vi "Conf_DO.vi"(8 "error in (no error)":errorcluster, 10 "PIN Number":i8, 11 "DI_DO in":refnum<class "DI_DO.lvclass">) -> (0 "error out":errorcluster, 3 "DI_DO out":refnum<class "DI_DO.lvclass">)   [LabVIEW 2023, in "Driver_DI_DO.lvlib" / "DI_DO.lvclass"]
uses:
  DI_DO.lvclass
  DI_DO.lvclass/DI_DO.ctl
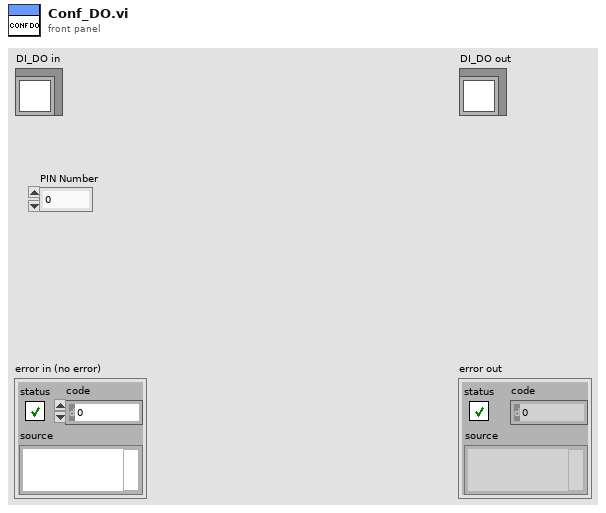
[diagram p1: front panel]
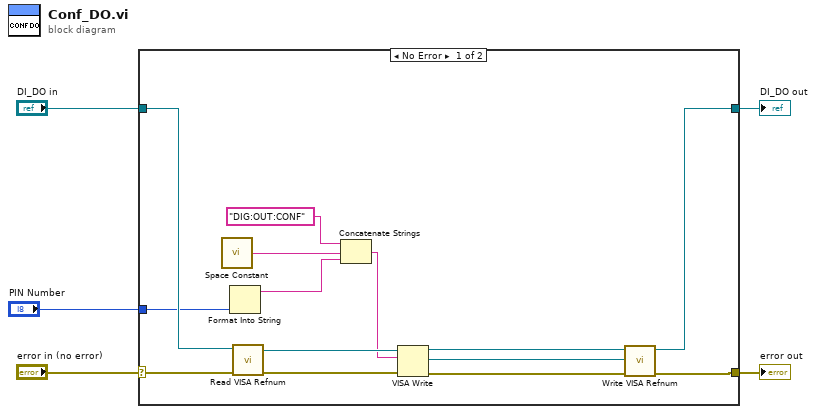
[diagram p0: block diagram]
diagram:
  n1 = case shown="No Error" "error in (no error)" {
    selector: "error in (no error)" -> [w18 w21]
    tunnel: [w9 w21] -> w4
    tunnel: [w7 w20] -> w2
    tunnel: "DI_DO in" -> [w19 w20]
    tunnel: "PIN Number" -> [w17 _]
    frame No Error {
      n2 = call <vilib>:"Space Constant.vi"() -> ("String"=w15:string)
      n3 = Format Into String(w17) -> (resulting string=w14:string)  [unwired: 3 in, 1 out]
      n4 = call-dynamic "Read VISA Refnum.vi"("error in (no error)"=w18, "Driver in"=w19) -> ("error out"=w11:errorcluster, "VISA Refnum"=w13:refnum<visa-resource-name>, "Driver out"=w6:refnum<class "DI_DO.lvclass">)  [unwired: 7 in]
      n5 = Concatenate Strings("DIG:OUT:CONF", w15, w14) -> (w12:string)
      n6 = VISA Write(VISA resource name=w13, write buffer=w12, error in (no error)=w11) -> (VISA resource name out=w8:refnum<visa-resource-name>, error out=w10:errorcluster)  [unwired: 1 out]
      n7 = call-dynamic "Write VISA Refnum.vi"("error in (no error)"=w10, "VISA Refnum"=w8, "Driver in"=w6) -> ("error out"=w9:errorcluster, "Driver out"=w7:refnum<class "DI_DO.lvclass">)  [unwired: 7 in]
    }
    frame Error {
    }
  }
  "error out" <- w4
  "DI_DO out" <- w2
